vi "SSL_set_fd.vi"(8 "error in (no error)":errorcluster, 10 "fd":u64, 11 "SSL in":refnum<class "SSL.lvclass">) -> (0 "error out":errorcluster, 3 "SSL out":refnum<class "SSL.lvclass">)   [LabVIEW 2013, in "OpenSSL Socket.lvlib" / "SSL.lvclass"]
uses:
  SSL.lvclass
  SSL-Lib/SSL-Lib.lvclass/SSL-Lib.ctl
  SSL.lvclass/SSL.ctl
  SSL-Lib/Read SSL Library Path.vi
  Read Handle.vi
  SSL-Lib/SSL-Lib.lvclass
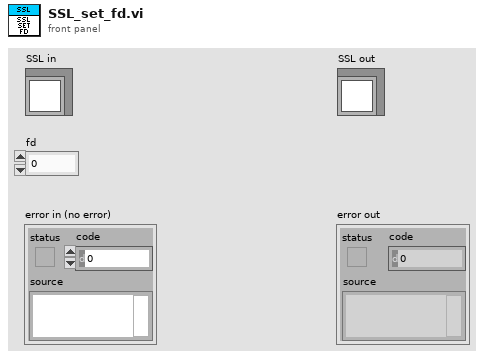
[diagram p1: front panel]
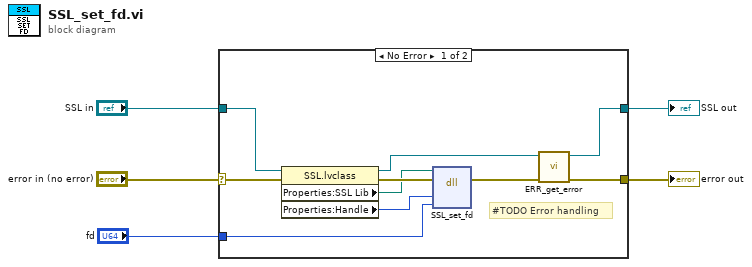
[diagram p0: block diagram]
diagram:
  n1 = case shown="No Error" "error in (no error)" {
    selector: "error in (no error)" -> [w15 w17]
    tunnel: [w9 w17] -> w4
    tunnel: [w7 w16] -> w2
    tunnel: "SSL in" -> [w6 w16]
    tunnel: "fd" -> [w13 _]
    frame No Error {
      # "#TODO Error handling"
      n2 = property class="SSL.lvclass"(reference=w6, error in=w15) -> (reference out=w8:refnum<class "SSL.lvclass">, error out=w12:errorcluster, "Properties:SSL Lib"=w10:path, "Properties:Handle"=w11:u64)
      n3 = dll-call lib="C:/Program Files (x86)/National Instruments/Shared/nissl/NIssleay32.dll" fn="SSL_set_fd"(path in=w10, error in=w12, "*SSL"=w11, "fd"=w13) -> (error out=w14:errorcluster)  [unwired: 4 in, 1 out]
      n4 = call "ERR_get_error.vi"("error in (no error)"=w14, "SSL-Lib in"=w8) -> ("error out"=w9:errorcluster, "SSL-Lib out"=w7:refnum<class "SSL.lvclass">)  [unwired: 8 in]
    }
    frame Error {
    }
  }
  "error out" <- w4
  "SSL out" <- w2
